vi "Log.vi"(8 "error in (no error)":errorcluster, 10 "Message":string, 11 "Logger in":refnum<class "Logger.lvclass">) -> (0 "error out":errorcluster, 3 "Logger out":refnum<class "Logger.lvclass">)   [LabVIEW 2013, in "Logger.lvclass"]
doc: "Sends data (<string> \"Message\") to the Logger Object to be written a log (text) file by a background process.\n\nJared Kirschner, 2012."
uses:
  Logger.lvclass
  Logger.lvclass/Logger.ctl
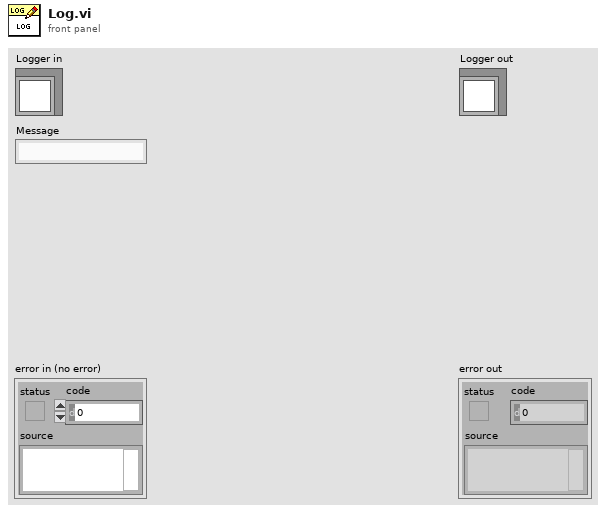
[diagram p1: front panel]
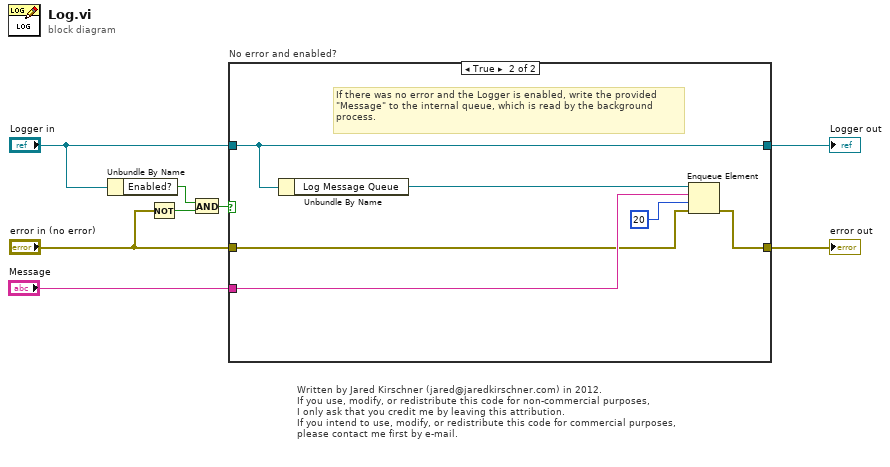
[diagram p0: block diagram]
diagram:
  # "Written by Jared Kirschner (jared@jaredkirschner.com) in 2012.\nIf you use, modify, or redistribute this code for non-commercial purposes,\nI only ask that you credit me by leaving this attribution.\nIf you intend to use, modify, or redistribute this code for commercial purposes,\nplease contact me first by e-mail."
  n1 = Unbundle By Name("Logger in") -> ("Enabled?"=w3:bool)
  n2 = Not(x="error in (no error)") -> (.not. x?=w2:bool)
  n3 = And(x=w3, y=w2) -> (x .and. y?=w4:bool)
  n4 = case "No error and enabled?" shown="True" w4 {
    tunnel: [w9 w13] -> w8
    tunnel: [w10 w16] -> w7
    tunnel: "Logger in" -> [w10 w16]
    tunnel: "Message" -> [_ w12]
    tunnel: "error in (no error)" -> [w9 w11]
    frame False {
      # "If there is an error or the logger was\nnot enabled in the initialize method,\ndo not log the data."
    }
    frame True {
      # "If there was no error and the Logger is enabled, write the provided\n\"Message\" to the internal queue, which is read by the background\nprocess."
      n5 = Unbundle By Name(w16) -> ("Log Message Queue"=w15:refnum<queue>)
      n6 = Enqueue Element(queue=w15, element=w12, timeout in ms (-1)=20, error in (no error)=w11) -> (error out=w13:errorcluster)  [unwired: 2 out]
    }
  }
  "error out" <- w8
  "Logger out" <- w7
